vi "GDSLvClass_StoreClassType.vi"(0 "Class Refnum In":refnum<vi>, 1 "ClassSettings":T1, 3 "CheckAndFixConnectorPaneType(False)":bool, 5 "error in (no error)":errorcluster) -> (14 "Class Refnum Out":refnum<vi>, 19 "error out":errorcluster)   [LabVIEW 2020]
uses:
  <resource>/Framework/Providers/Open_GDS/ClassProviders/Common/LvClass_class/GDSLvCLass_ClassSettingsType.ctl
  <resource>/Framework/Providers/Open_GDS/ClassProviders/Common/LvClass_class/GDSLvClass_PlugIn.ctl
  <resource>/Framework/Providers/Open_GDS/ClassProviders/Common/LvClass_class/GDSLvClass_PlugInTypes.ctl
  <resource>/Framework/Providers/Open_GDS/ClassProviders/Common/LvClass_class/GDSLvClass_ClassTypeSettingNames.ctl
  <resource>/Framework/Providers/Open_GDS/ClassProviders/Common/ScriptingFunctions/Scripting_ConnectorPanePatternType.ctl
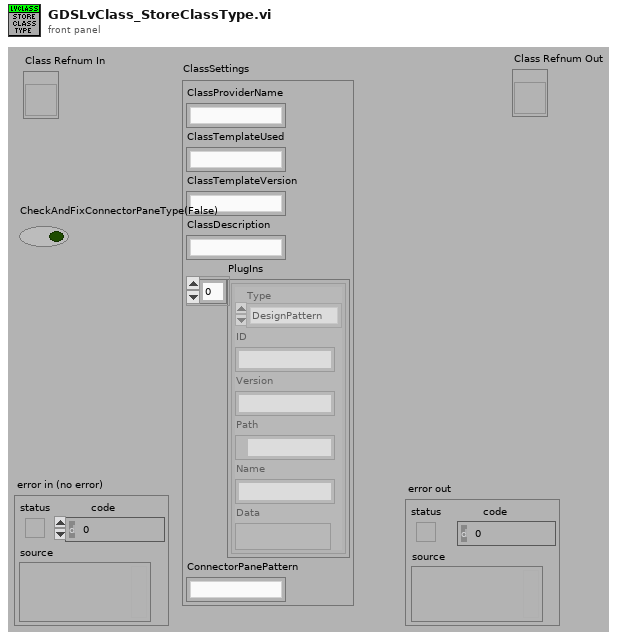
[diagram p1: front panel]
types:
  T1 = typedef "GDSLvCLass_ClassSettingsType.ctl" = cluster{"ClassProviderName":string, "ClassTemplateUsed":string, "ClassTemplateVersion":string, "ClassDescription":string, "PlugIns":T2[], "ConnectorPanePattern":string}
  T2 = typedef "GDSLvClass_PlugIn.ctl" = cluster{"Type":T3, "ID":string, "Version":string, "Path":path, "Name":string, "Data":variant}
  T3 = typedef "GDSLvClass_PlugInTypes.ctl" = enum16{"DesignPattern", "MethodTypes"}
  T4 = typedef "GDSLvClass_ClassTypeSettingNames.ctl" = enum16{"EndevoGOOP_ClassProvider", "EndevoGOOP_TemplateUsed", "EndevoGOOP_TemplateVersion", "EndevoGOOP_PlugIns", "EndevoGOOP_ConnectorPanePattern"}
  T5 = typedef "Scripting_ConnectorPanePatternType.ctl" = u16
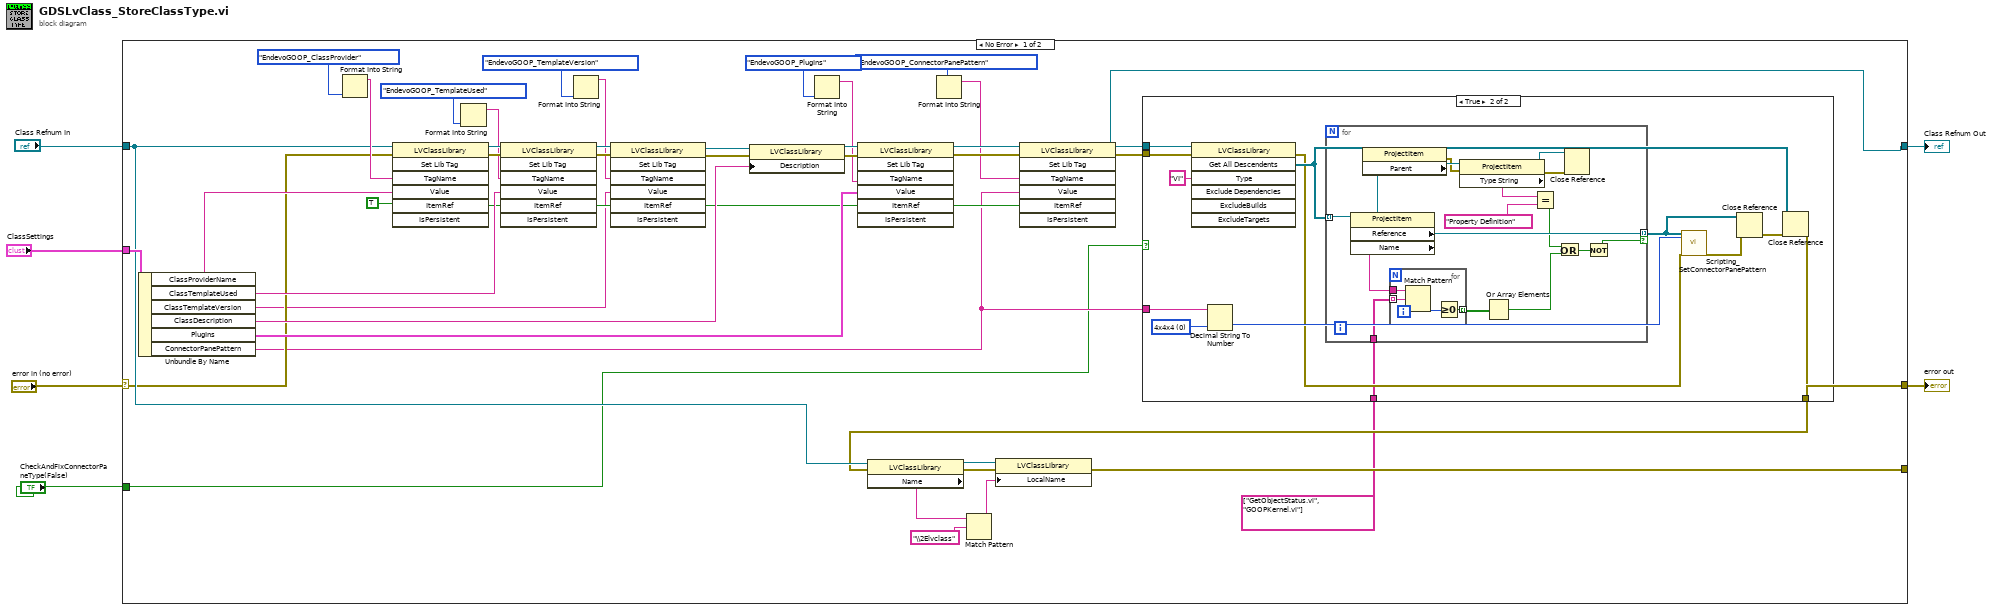
[diagram p0: block diagram]
diagram:
  n1 = case shown="No Error" "error in (no error)" {
    selector: "error in (no error)" -> [w20 w83]
    tunnel: [w10 w83] -> w5
    tunnel: "Class Refnum In" -> [w21 w82]
    tunnel: [w8 w82] -> w3
    tunnel: "ClassSettings" -> [w35 _]
    tunnel: [w13 _] -> _
    tunnel: "CheckAndFixConnectorPaneType(False)" -> [w9 _]
    frame No Error {
      w22 = TRUE ("Is Persistent")
      n2 = Unbundle By Name(w35) -> ("ClassProviderName"=w34:string, "ClassTemplateUsed"=w33:string, "ClassTemplateVersion"=w19:string, "ClassDescription"=w32:string, "PlugIns"=w29:T2[], "ConnectorPanePattern"=w12:string)
      n3 = Format Into String(GDSLvClass_ClassTypeSettingNames."EndevoGOOP_ClassProvider" ("ClassTypeSettingNames")) -> (resulting string=w40:string)  [unwired: 3 in, 1 out]
      n4 = invoke class="LVClassLibrary" method="Set Lib Tag"(reference=w21, error in=w20, "TagName"=w40, "Value"=w34, "ItemRef"=w22) -> (reference out=w47:refnum<vi>, error out=w46:errorcluster)  [unwired: 2 in, 5 out]
      n5 = Format Into String(GDSLvClass_ClassTypeSettingNames."EndevoGOOP_TemplateUsed" ("ClassTypeSettingNames")) -> (resulting string=w38:string)  [unwired: 3 in, 1 out]
      n6 = invoke class="LVClassLibrary" method="Set Lib Tag"(reference=w47, error in=w46, "TagName"=w38, "Value"=w33, "ItemRef"=w22) -> (reference out=w45:refnum<vi>, error out=w44:errorcluster)  [unwired: 2 in, 5 out]
      n7 = Format Into String(GDSLvClass_ClassTypeSettingNames."EndevoGOOP_TemplateVersion" ("ClassTypeSettingNames")) -> (resulting string=w36:string)  [unwired: 3 in, 1 out]
      n8 = invoke class="LVClassLibrary" method="Set Lib Tag"(reference=w45, error in=w44, "TagName"=w36, "Value"=w19, "ItemRef"=w22) -> (reference out=w43:refnum<vi>, error out=w42:errorcluster)  [unwired: 2 in, 5 out]
      n9 = property class="LVClassLibrary"(reference=w43, error in=w42, "Description"=w32) -> (reference out=w31:refnum<vi>, error out=w30:errorcluster)
      n10 = Format Into String(GDSLvClass_ClassTypeSettingNames."EndevoGOOP_PlugIns" ("ClassTypeSettingNames")) -> (resulting string=w27:string)  [unwired: 3 in, 1 out]
      n11 = invoke class="LVClassLibrary" method="Set Lib Tag"(reference=w31, error in=w30, "TagName"=w27, "Value"=w29, "ItemRef"=w22) -> (reference out=w25:refnum<vi>, error out=w24:errorcluster)  [unwired: 2 in, 5 out]
      n12 = Format Into String(GDSLvClass_ClassTypeSettingNames."EndevoGOOP_ConnectorPanePattern" ("ClassTypeSettingNames")) -> (resulting string=w23:string)  [unwired: 3 in, 1 out]
      n13 = invoke class="LVClassLibrary" method="Set Lib Tag"(reference=w25, error in=w24, "TagName"=w23, "Value"=w12, "ItemRef"=w22) -> (reference out=w8:refnum<vi>, error out=w11:errorcluster)  [unwired: 2 in, 5 out]
      n14 = case shown="True" w9 {
        tunnel: w8 -> [_ w61]
        tunnel: w12 -> [_ w59]
        tunnel: w11 -> [w48 w52]
        tunnel: [w48 w50] -> w10
        tunnel: string[] ["GetObjectStatus.vi", "GOOPKernel.vi"] -> [_ w49]
        frame False {
        }
        frame True {
          w58 = T5 0 items=["4x4x4", "5x6x5", "6x8x6"] ("Pattern")
          n15 = invoke class="LVClassLibrary" method="Get All Descendents"(reference=w61, error in=w52, "Type"="VI") -> (error out=w51:errorcluster, "All Descendents"=w53:refnum<vi>[])  [unwired: 4 in, 5 out]
          n16 = Decimal String To Number(string=w59, default (0L)=w58) -> (number=w57:u16)  [unwired: 1 in, 1 out]
          n17 = for {
            tunnel: w53 -> [w77] mode=indexing
            tunnel: [w72] -> w56 mode=indexing if=w73
            tunnel: w49 -> [w75]
            n18 = property class="ProjectItem"(reference=w77) -> (reference out=w71:refnum<vi>, "Reference"=w72:refnum<vi>, "Name"=w76:string)  [unwired: 1 in, 1 out]
            n19 = property class="ProjectItem"(reference=w71) -> (error out=w62:errorcluster, "Parent"=w70:refnum<vi>)  [unwired: 1 in, 1 out]
            n20 = for {
              tunnel: w76 -> [w81]
              tunnel: w75 -> [w80] mode=indexing
              tunnel: [w78] -> w74 mode=indexing
              n21 = Match Pattern(string=w81, regular expression=w80) -> (offset past match=w79:i32)  [unwired: 1 in, 3 out]
              n22 = Greater Or Equal To 0?(x=w79) -> (x >= 0?=w78:bool)
            }
            n23 = property class="ProjectItem"(reference=w70, error in=w62) -> (reference out=w64:refnum<vi>, error out=w63:errorcluster, "Type String"=w69:string)
            n24 = Or Array Elements(Boolean array=w74) -> (logical OR=w66:bool)
            n25 = Equal?(x=w69, y="Property Definition") -> (x = y?=w67:bool)
            n26 = Or(x=w67, y=w66) -> (x .or. y?=w65:bool)
            n27 = Close Reference(reference=w64, error in (no error)=w63) -> ()  [unwired: 1 out]
            n28 = Not(x=w65) -> (.not. x?=w73:bool)
          }
          n29 = call <resource>:"Scripting_SetConnectorPanePattern.vi"("VIPath(s)/ViRef(s)"=w56, "Pattern"=w57, "error in (no error)"=w51) -> ("error out"=w55:errorcluster)  [unwired: 16 in]
          n30 = Close Reference(reference=w56, error in (no error)=w55) -> (error out=w54:errorcluster)
          n31 = Close Reference(reference=w53, error in (no error)=w54) -> (error out=w50:errorcluster)
        }
      }
      n32 = property class="LVClassLibrary"(reference=w21, error in=w10) -> (reference out=w18:refnum<vi>, error out=w17:errorcluster, "Name"=w16:string)
      n33 = Match Pattern(string=w16, regular expression="\\2Elvclass") -> (before substring=w14:string)  [unwired: 1 in, 3 out]
      n34 = property class="LVClassLibrary"(reference=w18, error in=w17, "LocalName"=w14) -> (error out=w13:errorcluster)  [unwired: 1 out]
    }
    frame Error {
    }
  }
  "Class Refnum Out" <- w3
  "error out" <- w5
